vi "LJM logger startup config.vi"(7 "Device Open Config Name":string="openconfig.cfg", 8 "Program Config Name":string="expconfig.cfg", 9 "Working Directory":path) -> (1 "Open Config Identifier":string, 2 "Open Config ConnectionType":string, 3 "Open Config Device Type":string, 4 "Program Configs":T1={"Data File Prefix"="", "Scan Rate (Hz)"=0.0, "Graph History"=0, "# Channels"=0, "Disable Scaling"=FALSE, "Max File Size (Bytes)"=0, "Channel Setup"={"Name"=["AIN0", "AIN1", "AIN2", "AIN3", "AIN4", "AIN5", "AIN6", "AIN7", "AIN8", "AIN9", "AIN10", "AIN11", "AIN12", "AIN13", "AIN14", "AIN15"], "", "Scaling Equation"=["y=a", "y=b", "y=c", "y=d", "y=e", "y=f", "y=g", "y=h", "y=i", "y=j", "y=k", "y=l", "y=m", "y=n", "y=o", "y=p"], "", "Graph?"=[TRUE, TRUE, TRUE, TRUE, FALSE, FALSE, FALSE, FALSE, FALSE, FALSE, FALSE, FALSE, FALSE, FALSE, FALSE, FALSE]}, "Interval (ms)"=0, "Write To File"=FALSE, "Log Every n Scans"=0})   [LabVIEW 2026]
uses:
  Common Logger Controls/Program Config Cluster.ctl
  Common Logger Controls/Channel Setup.ctl
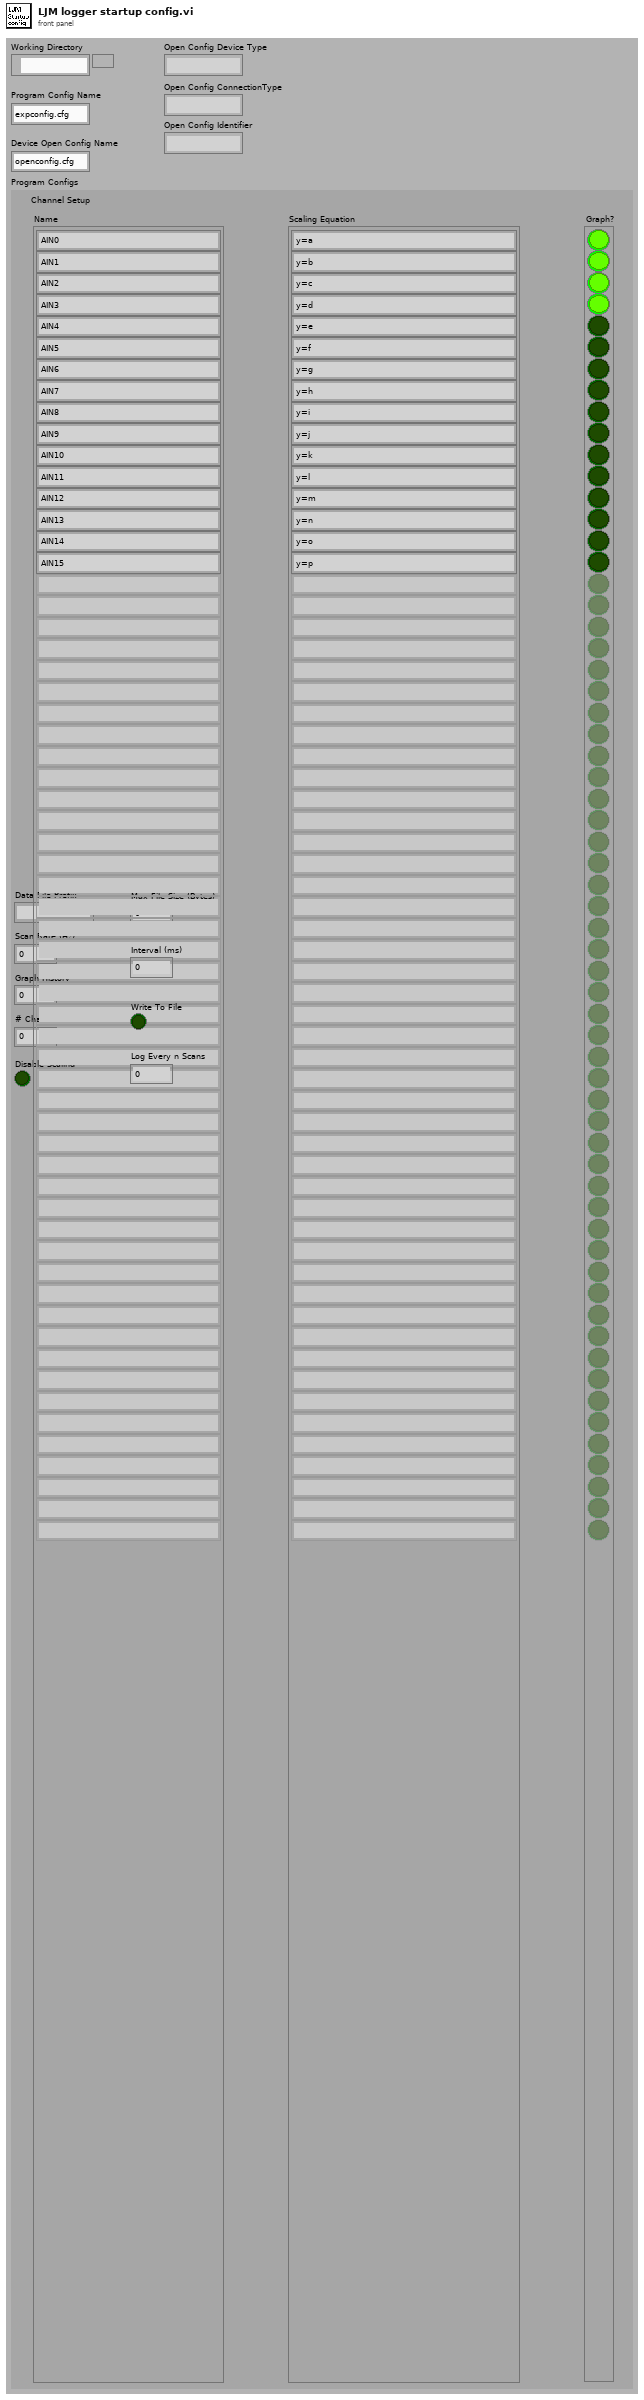
[diagram p1: front panel]
types:
  T1 = typedef "Program Config Cluster.ctl" = cluster{"Data File Prefix":string, "Scan Rate (Hz)":dbl, "Graph History":i32, "# Channels":i32, "Disable Scaling":bool, "Max File Size (Bytes)":i32, "Channel Setup":T2, "Interval (ms)":u32, "Write To File":bool, "Log Every n Scans":i32}
  T2 = typedef "Channel Setup.ctl" = cluster{"Name":string[], string, "Scaling Equation":string[], string, "Graph?":bool[]}
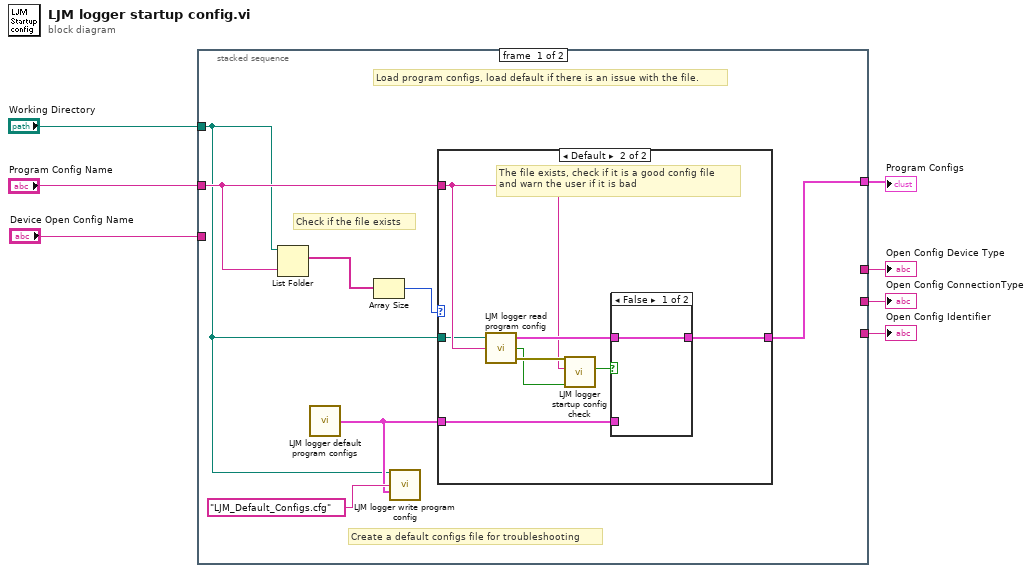
[diagram p0: block diagram]
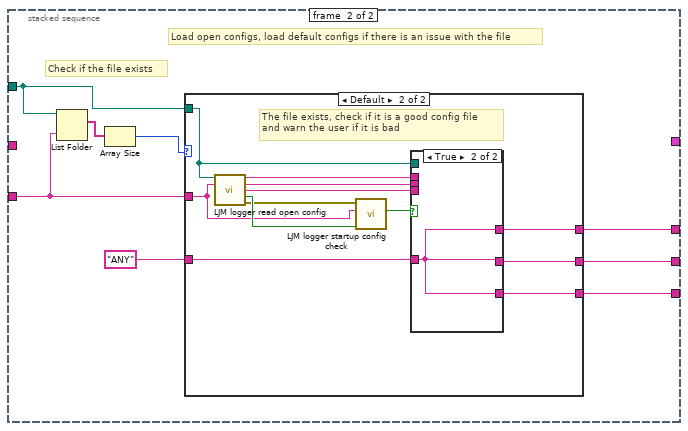
[diagram p4: hidden frame]
diagram:
  n1 = stacked-sequence {
    tunnel: [w14 _] -> w1
    tunnel: "Working Directory" -> [w9 w30]
    tunnel: "Program Config Name" -> [w10 _]
    tunnel: [_ w33] -> w6
    tunnel: [_ w32] -> w5
    tunnel: [_ w31] -> w4
    tunnel: "Device Open Config Name" -> [_ w29]
    frame #0 {
      # "Check if the file exists"
      # "Create a default configs file for troubleshooting"
      # "Load program configs, load default if there is an issue with the file."
      n2 = List Folder(path=w9, pattern=w10) -> (filenames=w11:string[])  [unwired: 2 in, 3 out]
      n3 = call "LJM logger default program configs.vi"() -> ("Program Configs"=w12:T1)  [unwired: 1 in]
      n4 = Array Size(array=w11) -> (size(s)=w8:i32)
      n5 = call "LJM logger write program config.vi"("Working Directory"=w9, "filename"="LJM_Default_Configs.cfg", "Program Configs"=w12) -> ()  [unwired: 12 in, 1 out]
      n6 = case shown="Default" w8 {
        tunnel: [w15 w20] -> w14
        tunnel: w12 -> [w15 w18]
        tunnel: w10 -> [_ w17]
        tunnel: w9 -> [_ w16]
        frame 0 {
          # "File does not exist. Use the default configs"
        }
        frame Default {
          # "The file exists, check if it is a good config file\nand warn the user if it is bad"
          n7 = call "LJM logger read program config.vi"("filename"=w17, "Working Directory"=w16) -> ("error out"=w22:errorcluster, "Good Program Config"=w21:bool, "Program Configs Out"=w19:T1)  [unwired: 1 in]
          n8 = call "LJM logger startup config check.vi"("Good Config?"=w21, "Config Name"=w17, "Config Error In"=w22) -> ("Force Defaults"=w23:bool)  [unwired: 8 in]
          n9 = case shown="False" w23 {
            tunnel: [w24 w25] -> w20
            tunnel: w19 -> [w24 _]
            tunnel: w18 -> [_ w25]
            frame False {
            }
            frame True {
            }
          }
        }
      }
    }
    frame #1 {
      # "Check if the file exists"
      # "Load open configs, load default configs if there is an issue with the file"
      n10 = List Folder(path=w30, pattern=w29) -> (filenames=w28:string[])  [unwired: 2 in, 3 out]
      n11 = Array Size(array=w28) -> (size(s)=w27:i32)
      n12 = case shown="Default" w27 {
        tunnel: [w34 w40] -> w33
        tunnel: [w34 w39] -> w32
        tunnel: [w34 w38] -> w31
        tunnel: w30 -> [_ w37]
        tunnel: w29 -> [_ w36]
        tunnel: "ANY" ("DeviceType") -> [w34 w35]
        frame 0 {
          # "File does not exist. Use the default configs"
        }
        frame Default {
          # "The file exists, check if it is a good config file\nand warn the user if it is bad"
          n13 = call "LJM logger read open config.vi"("Working Directory"=w37, "filename"=w36) -> ("Open Config Device Type"=w43:string, "Open Config Connection Type"=w42:string, "Open Config Identifier"=w41:string, "Good Open Config"=w46:bool, "error out"=w45:errorcluster)  [unwired: 9 in]
          n14 = call "LJM logger startup config check.vi"("Good Config?"=w46, "Config Name"=w36, "Config Error In"=w45) -> ("Force Defaults"=w44:bool)  [unwired: 8 in]
          n15 = case shown="True" w44 {
            tunnel: w43 -> [w47 _]
            tunnel: w42 -> [w48 _]
            tunnel: w41 -> [w49 _]
            tunnel: w37 -> [_ _]
            tunnel: [w47 w50] -> w40
            tunnel: [w48 w50] -> w39
            tunnel: [w49 w50] -> w38
            tunnel: w35 -> [_ w50]
            frame False {
            }
            frame True {
            }
          }
        }
      }
    }
  }
  "Open Config Device Type" <- w6
  "Open Config ConnectionType" <- w5
  "Open Config Identifier" <- w4
  "Program Configs" <- w1
